vi "Get All Items By Enumerator.vi"(8 "error in (no error)":errorcluster caption="错误输入（无错误）", 11 "ArrayListClass 输入":refnum<class "ArrayListClass.lvclass"> caption="DNL_LabVIEW Object in") -> (0 "error out":errorcluster caption="错误输出", 2 "Items":variant[](array[variant]), 3 "ArrayListClass 输出":refnum<class "ArrayListClass.lvclass"> caption="DNL_LabVIEW Object out")   [LabVIEW 2012, in "ArrayListClass.lvclass"]
uses:
  ArrayListClass.lvclass
  Enumerator/Enumerator.lvclass
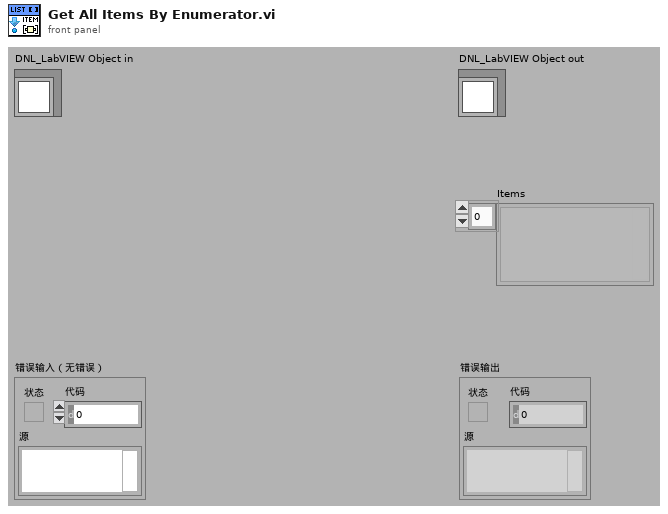
[diagram p1: front panel]
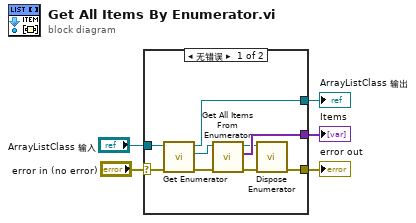
[diagram p0: block diagram]
diagram:
  n1 = case shown="无错误" "error in (no error)" {
    selector: "error in (no error)" -> [w12 w16]
    tunnel: [w6 w16] -> w4
    tunnel: [w11 w15] -> w2
    tunnel: "ArrayListClass 输入" -> [w13 w15]
    tunnel: [w14 _] -> w1
    frame No Error {
      n2 = call "Get Enumerator.vi"("error in (no error)"=w12, "ArrayListClass 输入"=w13) -> ("error out"=w9:errorcluster, "Enumerator 输出"=w10:refnum<class "Enumerator.lvclass">, "ArrayListClass 输出"=w11:refnum<class "ArrayListClass.lvclass">)  [unwired: 7 in]
      n3 = call "Get All Items From Enumerator.vi"("error in (no error)"=w9, "Enumerator 输入"=w10) -> ("error out"=w8:errorcluster, "Items"=w14:variant[], "Enumerator 输出"=w7:refnum<class "Enumerator.lvclass">)  [unwired: 7 in]
      n4 = call "Dispose Enumerator.vi"("error in (no error)"=w8, "Enumerator 输入"=w7) -> ("error out"=w6:errorcluster)  [unwired: 8 in, 1 out]
    }
    frame Error {
    }
  }
  "error out" <- w4
  "ArrayListClass 输出" <- w2
  "Items" <- w1
